vi "FTW-Endpoint-Multipart-Reply.vi"(0 "FTW Endpoint":refnum<class "FTW-Endpoint-TCP.lvclass">, 5 "Message":T1, 7 "Timeout":i32 format="%dmsec", 11 "error in":errorcluster) -> (4 "FTW Endpoint out":refnum<class "FTW-Endpoint-TCP.lvclass">, 6 "Timed out?":bool, 15 "error out":errorcluster)   [LabVIEW 2013, in "FTW-Endpoint-TCP.lvclass"]
uses:
  FTW-Endpoint-TCP.lvclass
  Message/FTW-Message.ctl
  FTW-Endpoint-TCP.lvclass/FTW-Endpoint-TCP.ctl
  Error/FTW-ERR-Clear.vi
panel:
  # "Inputs"
  # "Outputs"
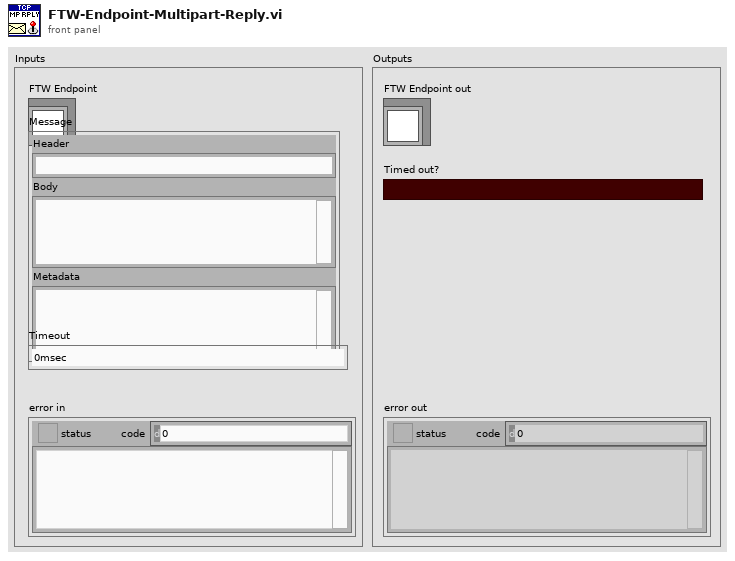
[diagram p1: front panel]
types:
  T1 = typedef "FTW-Message.ctl" = cluster{"Header":string, "Body":string, "Metadata":string}
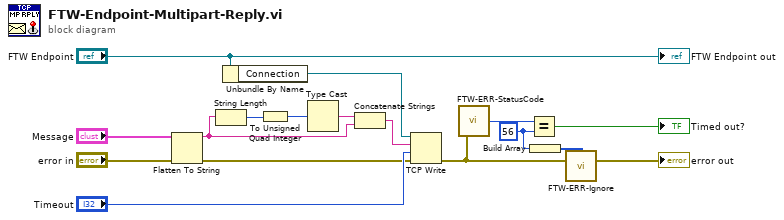
[diagram p0: block diagram]
diagram:
  w3 = 56 ("x")
  n1 = Flatten To String(anything="Message", error in (no error)="error in") -> (data string=w4:string, error out=w11:errorcluster)  [unwired: 2 in, 1 out]
  n2 = String Length(string=w4) -> (length=w7:i32)
  n3 = Unbundle By Name("FTW Endpoint") -> ("Connection"=w10:refnum<k5>)
  n4 = To Unsigned Quad Integer(1:w7) -> (0:w1:u64)
  n5 = Type Cast(x=w1) -> (*(type *) &x=w6:string)  [unwired: 1 in]
  n6 = Concatenate Strings(w6, w4) -> (w5:string)
  n7 = TCP Write(connection ID=w10, data in=w5, error in (no error)=w11, 9:"Timeout") -> (error out=w9:errorcluster)  [unwired: 2 out]
  n8 = call "FTW-ERR-StatusCode.vi"("error to check"=w9) -> ("Code"=w8:i32)
  n9 = Equal?(x=w8, y=w3) -> (x = y?=→"Timed out?":bool)
  n10 = Build Array(w3) -> (w2:i32[])
  n11 = call "FTW-ERR-Ignore.vi"("Codes to filter"=w2, "error to filter"=w9) -> ("filtered error"=→"error out":errorcluster)  [unwired: 13 in]
  "FTW Endpoint out" <- "FTW Endpoint"
